vi "Set Acquisition Configuration.vi"(8 "error in (no error)":errorcluster, 11 "CCDCamera in":refnum<class "iKon-L.lvclass">) -> (0 "error out":errorcluster, 3 "CCDCamera out":refnum<class "iKon-L.lvclass">)   [LabVIEW 2018, in "iKon-L.lvclass"]
doc: "Set the camera configuration\n\nThis function records the given operating parameters in the camera. However, the parameters will only bewritten if their last value is different from the most recent one."
uses:
  iKon-L.lvclass
  C:/Users/Denis/Desktop/S4ACS/S4ACS/Sim_CCD/Sim_CCD.lvclass
  Sim_CCD/Sim_CCD.lvclass
panel:
  out "x != y?":T1
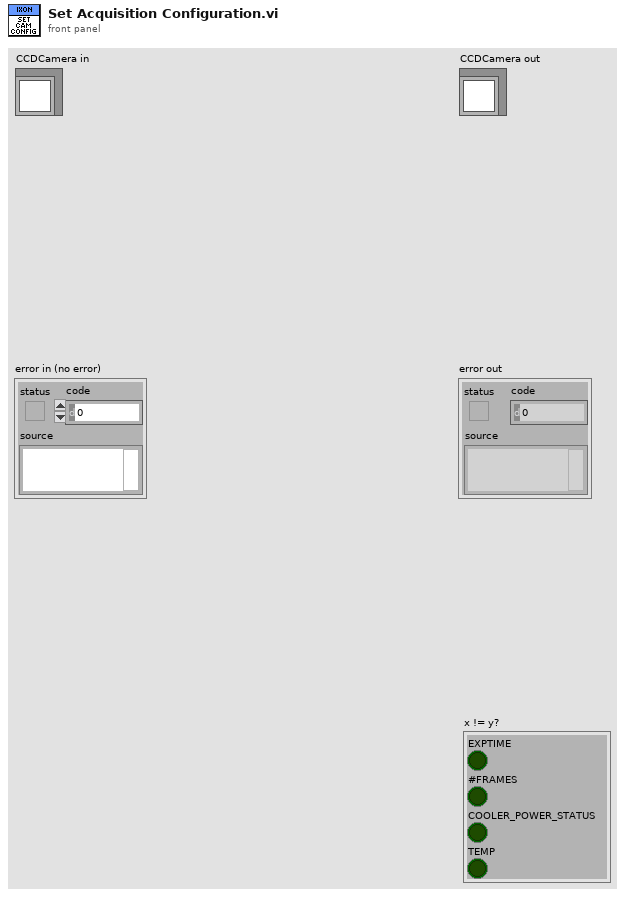
[diagram p1: front panel]
types:
  T1 = cluster{"EXPTIME":bool, "#FRAMES":bool, "COOLER_POWER_STATUS":bool, "TEMP":bool}
  T2 = cluster{"EXPTIME":dbl, "#FRAMES":u32, "COOLER_POWER_STATUS":u16, "TEMP":i32}
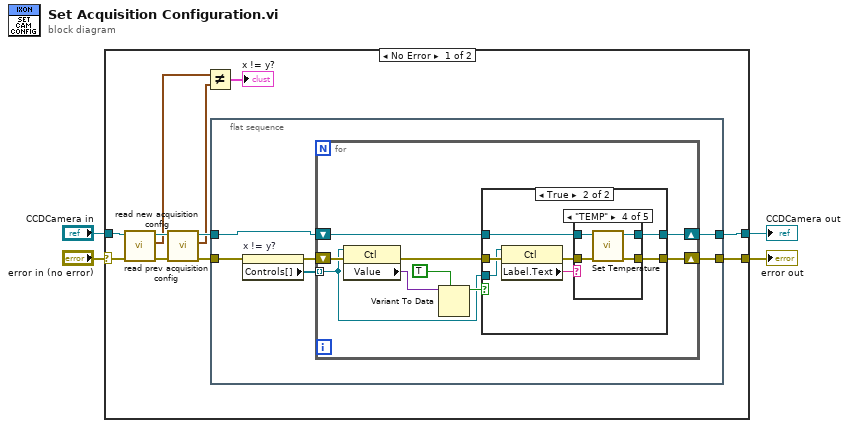
[diagram p0: block diagram]
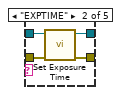
[diagram p4: hidden frame]
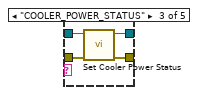
[diagram p5: hidden frame]
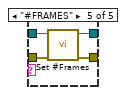
[diagram p6: hidden frame]
diagram:
  n1 = case shown="No Error" "error in (no error)" {
    selector: "error in (no error)" -> [w12 w59]
    tunnel: [w15 w59] -> w4
    tunnel: [w14 w58] -> w3
    tunnel: "CCDCamera in" -> [w13 w58]
    frame No Error {
      n2 = call "read prev acquisition config.vi"("error in (no error)"=w12, "Simulated_CCD_Camera in"=w13) -> ("error out"=w8:errorcluster, "prev acquisition configuration"=w7:T2, "Simulated_CCD_Camera out"=w11:refnum<class "iKon-L.lvclass">)  [unwired: 7 in]
      n3 = call "read new acquisition config.vi"("error in (no error)"=w8, "Simulated_CCD_Camera in"=w11) -> ("error out"=w9:errorcluster, "new acquisition configuration"=w6:T2, "Simulated_CCD_Camera out"=w10:refnum<class "iKon-L.lvclass">)  [unwired: 7 in]
      n4 = Not Equal?(x=w7, y=w6) -> (x != y?=→"x != y?":T1)
      n5 = flat-sequence {
        tunnel: w9 -> [w17]
        tunnel: [w21] -> w15
        tunnel: w10 -> [w20]
        tunnel: [w19] -> w14
        frame #0 {
          n6 = property on="x != y?" class="Clust (strict)"(error in=w17) -> (error out=w16:errorcluster, "Controls[]"=w18:refnum<vi>[])  [unwired: 1 in, 1 out]
          n7 = for {
            shift-right: [w25] -> w21
            shift-left: w16 -> [w24]
            shift-right: [w26] -> w19
            shift-left: w20 -> [w27]
            tunnel: w18 -> [w22] mode=indexing
            n8 = property class="Ctl"(reference=w22, error in=w24) -> (error out=w23:errorcluster, "Value"=w30:variant)  [unwired: 1 out]
            n9 = Variant To Data(type=TRUE, Variant=w30) -> (data=w28:bool)  [unwired: 1 in, 1 out]
            n10 = case shown="True" w28 {
              tunnel: [w32 w34] -> w25
              tunnel: w23 -> [w32 w38]
              tunnel: w27 -> [w31 w37]
              tunnel: [w31 w36] -> w26
              tunnel: w22 -> [_ w33]
              frame False {
              }
              frame True {
                n11 = property class="Ctl"(reference=w33, error in=w38) -> (error out=w35:errorcluster, "Label.Text"=w39:string)  [unwired: 1 out]
                n12 = case shown="\"TEMP\"" w39 {
                  tunnel: w37 -> [w41 w45 w48 w50 w56]
                  tunnel: [w41 w44 w47 w51 w57] -> w36
                  tunnel: w35 -> [w40 w43 w49 w53 w55]
                  tunnel: [w40 w42 w46 w52 w54] -> w34
                  frame "False", Default {
                  }
                  frame "EXPTIME" {
                    n13 = call-dynamic "Set Exposure Time.vi"("error in (no error)"=w43, "CCDCamera in"=w45) -> ("error out"=w42:errorcluster, "CCDCamera out"=w44:refnum<class "iKon-L.lvclass">)  [unwired: 8 in]
                  }
                  frame "COOLER_POWER_STATUS" {
                    n14 = call-dynamic "Set Cooler Power Status.vi"("error in (no error)"=w49, "CCDCamera in"=w48) -> ("error out"=w46:errorcluster, "CCDCamera out"=w47:refnum<class "iKon-L.lvclass">)  [unwired: 8 in]
                  }
                  frame "TEMP" {
                    n15 = call-dynamic "Set Temperature.vi"("error in (no error)"=w53, "CCDCamera in"=w50) -> ("error out"=w52:errorcluster, "CCDCamera out"=w51:refnum<class "iKon-L.lvclass">)  [unwired: 8 in]
                  }
                  frame "#FRAMES" {
                    n16 = call-dynamic "Set #Frames.vi"("error in (no error)"=w55, "CCDCamera in"=w56) -> ("error out"=w54:errorcluster, "CCDCamera out"=w57:refnum<class "iKon-L.lvclass">)  [unwired: 8 in]
                  }
                }
              }
            }
          }
        }
      }
    }
    frame Error {
    }
  }
  "error out" <- w4
  "CCDCamera out" <- w3
